vi "Functional Global - Queues.vi"(8 "Error In":errorcluster) -> (0 "Error Out":errorcluster, 1 "Data Q":refnum<queue>, 2 "Data Producer Control Q":refnum<queue>, 3 "Comsumer Events Data Q":refnum<queue>, 5 "Producer Consumer Events Q":refnum<queue>)   [LabVIEW 2014]
uses:
  Enum State Typedef.ctl
  Consumer Data_ Consumer Event Com.ctl
  Data Producer States.ctl
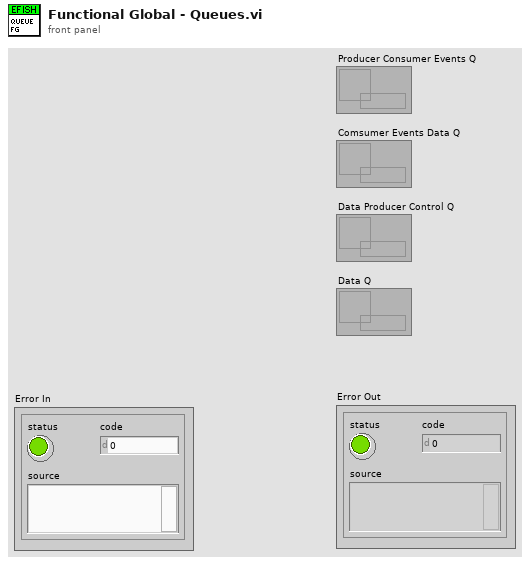
[diagram p1: front panel]
types:
  T1 = typedef "Data Producer States.ctl" = enum16{"Read Data", "Set Sample Clock", "Default", "Exit", "Preview"}
  T2 = typedef "Consumer Data_ Consumer Event Com.ctl" = enum16{"Recording", "Create File", "Clear Memory", "Default", "End File", "Exit", "Set Sample Clock", "Preview"}
  T3 = typedef "Enum State Typedef.ctl" = enum16{"Default", "Open FIle", "Beginning State", "Set the Sample Clock", "Prepreview Handling", "Clear Display", "Preview Data", "Stop", "Exit", "Record", "Create File"}
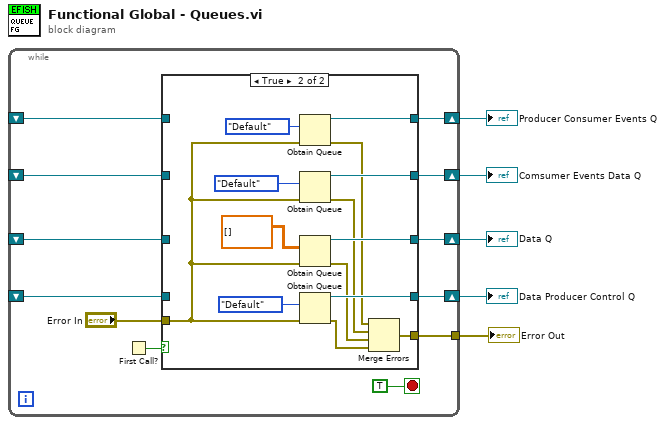
[diagram p0: block diagram]
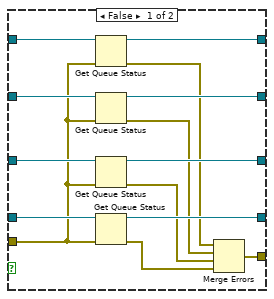
[diagram p2: hidden frame]
diagram:
  n1 = while {
    shift-right: [w15] -> w5
    shift-left: _ -> [w13]
    shift-right: [w14] -> w4
    shift-left: _ -> [w12]
    shift-right: [w11] -> w3
    shift-left: _ -> [w10]
    shift-right: [w9] -> w2
    shift-left: _ -> [w8]
    tunnel: [w7] -> w1
    stop <- TRUE stop-if-true
    n2 = First Call?() -> (First Call?: T/F=w17:bool)
    n3 = case shown="True" w17 {
      tunnel: [w24 w44] -> w15
      tunnel: [w25 w42] -> w14
      tunnel: w13 -> [w31 _]
      tunnel: w12 -> [w30 _]
      tunnel: [w26 w39] -> w11
      tunnel: w10 -> [w29 _]
      tunnel: [w27 w38] -> w9
      tunnel: w8 -> [w28 _]
      tunnel: [w23 w33] -> w7
      tunnel: "Error In" -> [w18 w32]
      frame False {
        n4 = Get Queue Status(queue=w31, error in (no error)=w18) -> (queue out=w24:refnum<queue>, error out=w22:errorcluster)  [unwired: 1 in, 6 out]
        n5 = Get Queue Status(queue=w30, error in (no error)=w18) -> (queue out=w25:refnum<queue>, error out=w21:errorcluster)  [unwired: 1 in, 6 out]
        n6 = Get Queue Status(queue=w29, error in (no error)=w18) -> (queue out=w26:refnum<queue>, error out=w20:errorcluster)  [unwired: 1 in, 6 out]
        n7 = Get Queue Status(queue=w28, error in (no error)=w18) -> (queue out=w27:refnum<queue>, error out=w19:errorcluster)  [unwired: 1 in, 6 out]
        n8 = Merge Errors(w22, w21, w20, w19) -> (w23:errorcluster)
      }
      frame True {
        n9 = Obtain Queue(element data type=Enum_State_Typedef."Default" ("State"), error in (no error)=w32) -> (queue out=w44:refnum<queue>, error out=w37:errorcluster)  [unwired: 3 in, 1 out]
        n10 = Obtain Queue(element data type=Consumer_Data__Consumer_Event_Com."Default", error in (no error)=w32) -> (queue out=w42:refnum<queue>, error out=w36:errorcluster)  [unwired: 3 in, 1 out]
        n11 = Obtain Queue(element data type=dbl[][] [], error in (no error)=w32) -> (queue out=w39:refnum<queue>, error out=w35:errorcluster)  [unwired: 3 in, 1 out]
        n12 = Obtain Queue(element data type=Data_Producer_States."Default", error in (no error)=w32) -> (queue out=w38:refnum<queue>, error out=w34:errorcluster)  [unwired: 3 in, 1 out]
        n13 = Merge Errors(w37, w36, w35, w34) -> (w33:errorcluster)
      }
    }
  }
  "Producer Consumer Events Q" <- w5
  "Comsumer Events Data Q" <- w4
  "Data Q" <- w3
  "Data Producer Control Q" <- w2
  "Error Out" <- w1
